vi "Test Morphology.vi"(8 "error in (no error)":errorcluster, 11 "Test Case In":refnum<class "01_Image.lvclass">) -> (0 "error out":errorcluster, 3 "Test Case Out":refnum<class "01_Image.lvclass">)   [LabVIEW 2020, in "test.lvlib" / "01_Image.lvclass"]
uses:
  01_Image.lvclass
  C:/Program Files (x86)/National Instruments/LabVIEW 2026/vi.lib/Astemes/LUnit/Test Case.lvclass
  common/Image Size (Integer).ctl
  <vilib>/Astemes/LUnit/Test Case.lvclass/Test Case.ctl
  ff8dbaef-6b31-4074-9b8a-3690e2ff7ea5.vi
  image/New Image (Greyscale Array).vi
  image/Get Morphology Structuring Element (Rectangle).vi
  image/New Image (Greyscale Preallocated).vi
  image/Morphology (Erode).vi
  image/Morphology (Dilate).vi
  image/Morphology (Gradient).vi
  image/Draw Image to Picture (Greyscale).vi
  500a0bd8-6df3-418a-afdb-164a7808fe68.vi
  image/MorphStructuringElementCore.vi
  image/New Image (Greyscale Preallocated).vi/6598b9e0-8a08-46f5-91fd-ca1b87217137.vi
  image/Copy Image (Greyscale).vi/c92252ab-1097-45af-a449-7a3c8cf05290.vi
  image/MorphologyCore.vi
  image/Draw Image to Picture (Greyscale).vi/9ae995ca-ccda-485c-89ac-02736fde3e8e.vi
  <vilib>/Astemes/LUnit/Core/LUnit Test Case/Private/Append Pass Result.vi
  <vilib>/Astemes/LUnit/Core/LUnit Test Case/Private/Append Fail Result.vi
  500a0bd8-6df3-418a-afdb-164a7808fe68.vi/9c5d11cd-9439-4240-a1ee-d9baace9c924.vi
  <vilib>/Astemes/LUnit/Core/LUnit Test Case/Private/Run In UI.vi
  <vilib>/Utility/error.llb/Clear Errors.vi
  <vilib>/Utility/error.llb/Error Cluster From Error Code.vi
  image/image.lvlib
  common/common.lvlib
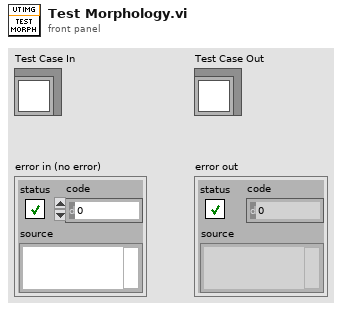
[diagram p1: front panel]
types:
  T1 = typedef "common.lvlib/Image Size (Integer).ctl" = cluster{"Width":u16, "Height":u16}
  T2 = typedef "image.lvlib/Greyscale Image.ctl" = refnum<data-value>
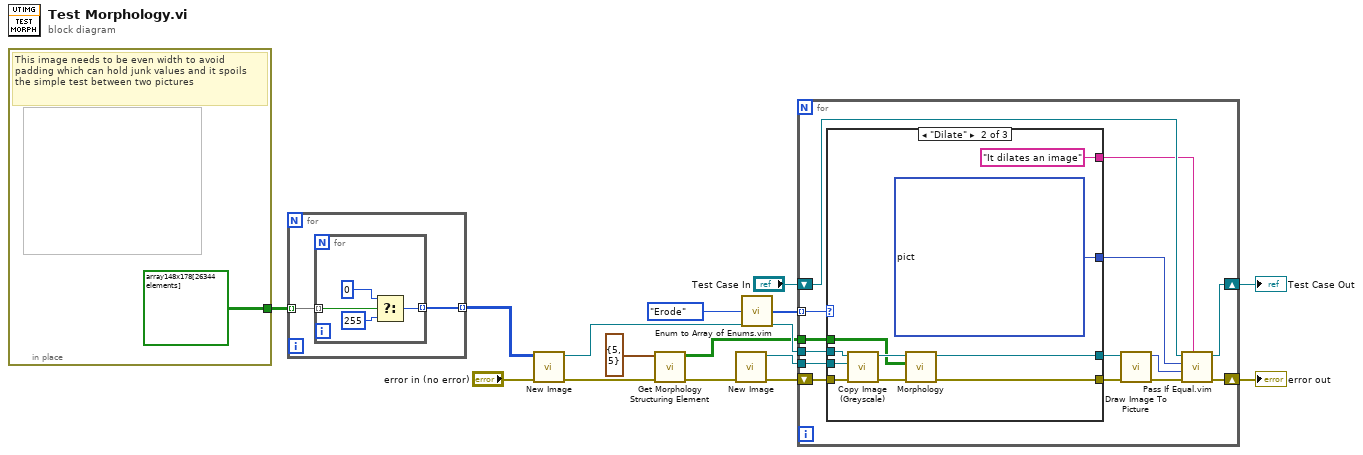
[diagram p0: block diagram]
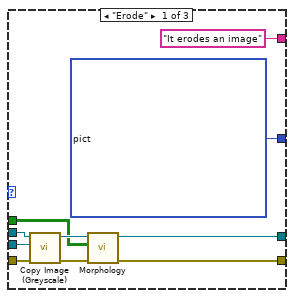
[diagram p2: hidden frame]
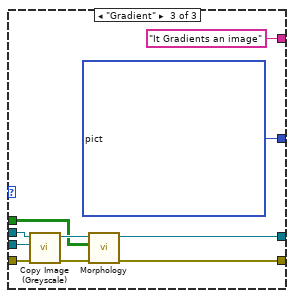
[diagram p3: hidden frame]
diagram:
  n1 = in-place {
    in-place-border: [bool[][] array148x178[26344 elements] ("1-bit pixmap")] -> w15
    # "This image needs to be even width to avoid padding which can hold junk values and it spoils the simple test between two pictures"
  }
  n2 = for {
    tunnel: w15 -> [w18] mode=indexing
    tunnel: [w17] -> w14 mode=indexing
    n3 = for {
      tunnel: w18 -> [w22] mode=indexing
      tunnel: [w20] -> w17 mode=indexing
      n4 = Select(t=u8 0, s=w22, f=u8 255) -> (s? t:f=w20:u8)
    }
  }
  n5 = call-poly "New Image.vi"("error in (no error)"="error in (no error)", "U8 Greyscale Data"=w14) -> ("error out"=w9:errorcluster, "Greyscale Image"=w13:T2)  [unwired: 8 in]
  n6 = call-poly "Get Morphology Structuring Element.vi"("error in (no error)"=w9, "Size"=T1 {"Width"=5, "Height"=5}) -> ("error out"=w8:errorcluster, "Structuring Element"=w11:bool[][])  [unwired: 8 in]
  n7 = call-poly "New Image.vi"("error in (no error)"=w8) -> ("error out"=w7:errorcluster, "Greyscale Image"=w12:T2)  [unwired: 9 in]
  n8 = call "Enum to Array of Enums.vim"("enum"=enum16{"Erode", "Dilate", "Gradient"}."Erode") -> ("array of enums"=w1:enum16{"Erode", "Dilate", "Gradient"}[])
  n9 = for {
    tunnel: w13 -> [w36]
    tunnel: w12 -> [w35]
    tunnel: w11 -> [w34]
    shift-right: [w29] -> w6
    shift-left: w7 -> [w33]
    shift-right: [w27] -> w3
    shift-left: "Test Case In" -> [w28]
    tunnel: w1 -> [w24] mode=indexing
    n10 = case shown="\"Dilate\"" w24 {
      tunnel: w36 -> [w40 w52 w59]
      tunnel: w35 -> [w39 w48 w58]
      tunnel: w34 -> [w37 w47 w57]
      tunnel: w33 -> [w46 w49 w62]
      tunnel: [w45 w56 w66] -> w32
      tunnel: [w44 w55 w65] -> w31
      tunnel: ["It erodes an image" ("Description") "It dilates an image" ("Description") "It Gradients an image" ("Description")] -> w26
      tunnel: [picture bytes[28424] ("Picture") picture bytes[28424] ("Picture") picture bytes[28424] ("Picture")] -> w25
      frame "Erode" {
        n11 = call "Copy Image (Greyscale).vi"("error in (no error)"=w46, "Greyscale Image Destination in"=w39, "Greyscale Image Source in"=w40) -> ("error out"=w41:errorcluster, "Greyscale Image Destination"=w38:T2)  [unwired: 7 in]
        n12 = call-poly "Morphology.vi"("error in (no error)"=w41, "Structuring Element"=w37, "Greyscale Image-Source in"=w38) -> ("error out"=w44:errorcluster, "Greyscale Image-Source"=w45:T2)  [unwired: 7 in]
      }
      frame "Dilate" {
        n13 = call "Copy Image (Greyscale).vi"("error in (no error)"=w49, "Greyscale Image Destination in"=w48, "Greyscale Image Source in"=w52) -> ("error out"=w50:errorcluster, "Greyscale Image Destination"=w51:T2)  [unwired: 7 in]
        n14 = call-poly "Morphology.vi"("error in (no error)"=w50, "Structuring Element"=w47, "Greyscale Image-Source in"=w51) -> ("error out"=w55:errorcluster, "Greyscale Image-Source"=w56:T2)  [unwired: 7 in]
      }
      frame "Gradient" {
        n15 = call "Copy Image (Greyscale).vi"("error in (no error)"=w62, "Greyscale Image Destination in"=w58, "Greyscale Image Source in"=w59) -> ("error out"=w61:errorcluster, "Greyscale Image Destination"=w60:T2)  [unwired: 7 in]
        n16 = call-poly "Morphology.vi"("error in (no error)"=w61, "Structuring Element"=w57, "Greyscale Image-Source in"=w60) -> ("error out"=w65:errorcluster, "Greyscale Image-Source"=w66:T2)  [unwired: 7 in]
      }
    }
    n17 = call-poly "Draw Image To Picture.vi"("error in (no error)"=w31, "Greyscale Image Source in"=w32) -> ("error out"=w30:errorcluster, "Picture"=w23:picture)  [unwired: 8 in]
    n18 = call "Pass If Equal.vim"("Description"=w26, "error in (no error)"=w30, "Actual"=w23, "Expected"=w25, "LUnit Test Case In"=w28) -> ("error out"=w29:errorcluster, "LUnit Test Case Out"=w27:refnum<class "01_Image.lvclass">)  [unwired: 5 in]
  }
  "error out" <- w6
  "Test Case Out" <- w3
